vi "Sequencer List Entry Move Up.vi"(8 "error in (no error)":errorcluster, 9 "Index (0)":i32, 10 "Instance (1)":i32=1, 11 "VISA resource name":refnum<visa-resource-name>) -> (0 "error out":errorcluster, 3 "VISA resource name out":refnum<visa-resource-name>)   [LabVIEW 2020, in "Rohde&Schwarz CMXP GPRF.lvlib"]
doc: "Moves the selected entry of the sequencer list one position up.\nThe selection moves with the entry.\n\nAttribute:\nRSCMXPGPRF_ATTR_SEQUENCER_LIST_ENTRY_MOVE_UP\n\nRemote-control command:\nSOURce:GPRF:GEN<i>:SEQuencer:LIST:ENTRy:MUP"
uses:
  <instrlib>/Rohde&Schwarz CMXP GPRF/Rohde&Schwarz CMXP GPRF.lvlib
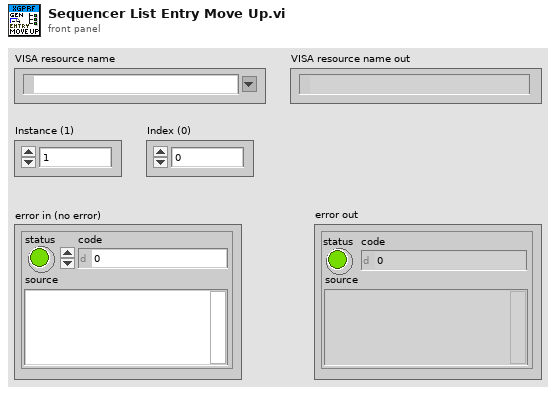
[diagram p1: front panel]
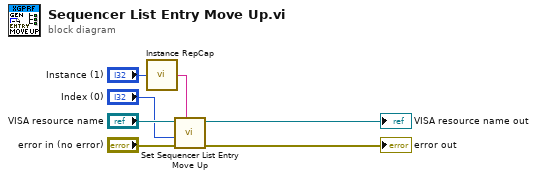
[diagram p0: block diagram]
diagram:
  n1 = call <instrlib>:"Instance RepCap.vi"("Instance in"="Instance (1)") -> ("Instance out"=w2:string)
  n2 = call "Set Sequencer List Entry Move Up"("Repeated Capabilities"=w2, "error in (no error)"="error in (no error)", "Sequencer List Entry Move Up (0)"="Index (0)", "instrument handle"="VISA resource name") -> ("error out"=→"error out":errorcluster, "instrument handle out"=→"VISA resource name out":refnum<visa-resource-name>)  [unwired: 6 in]
